vi "9401PWM with Midi.vi"() -> ()   [LabVIEW 2013]
panel:
  out "PWM1":dbl
  out "x .and. y?":bool
  out "error out 2":errorcluster
  out "duration (min:sec)":string="0:00"
  out "Text":string
  out "Track number: name [channel(s) used]":string="Please select a MIDI file..."
  in  "MIDI file (.mid)":path
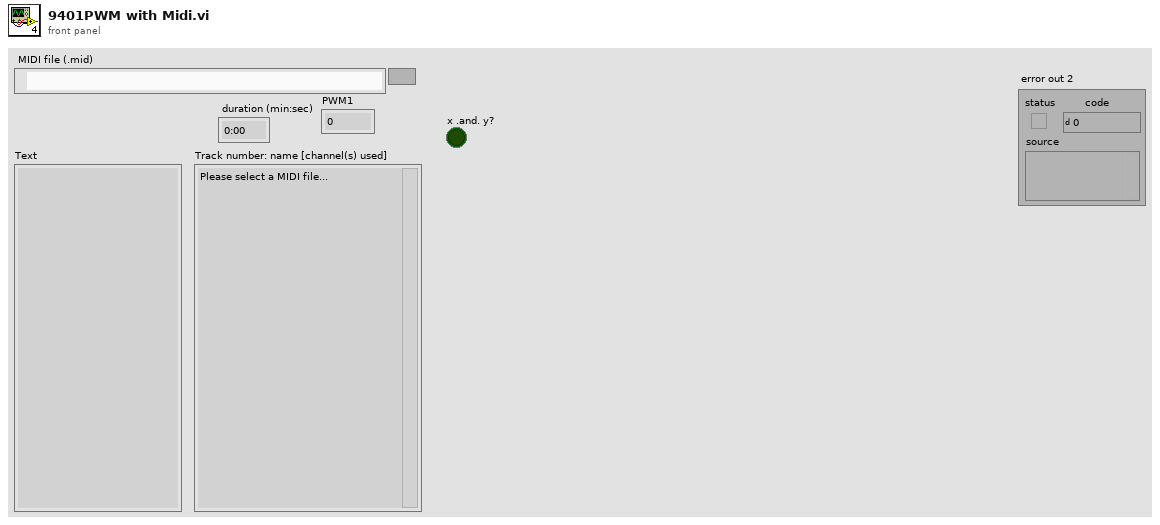
[diagram p1: front panel]
types:
  T1 = cluster{"type":u16, "tracks":u16, "ticks per qnote":u16}
  T2 = cluster{"note events":dbl[][], "duration [seconds]":dbl, "track info":string, "text meta-events":string}
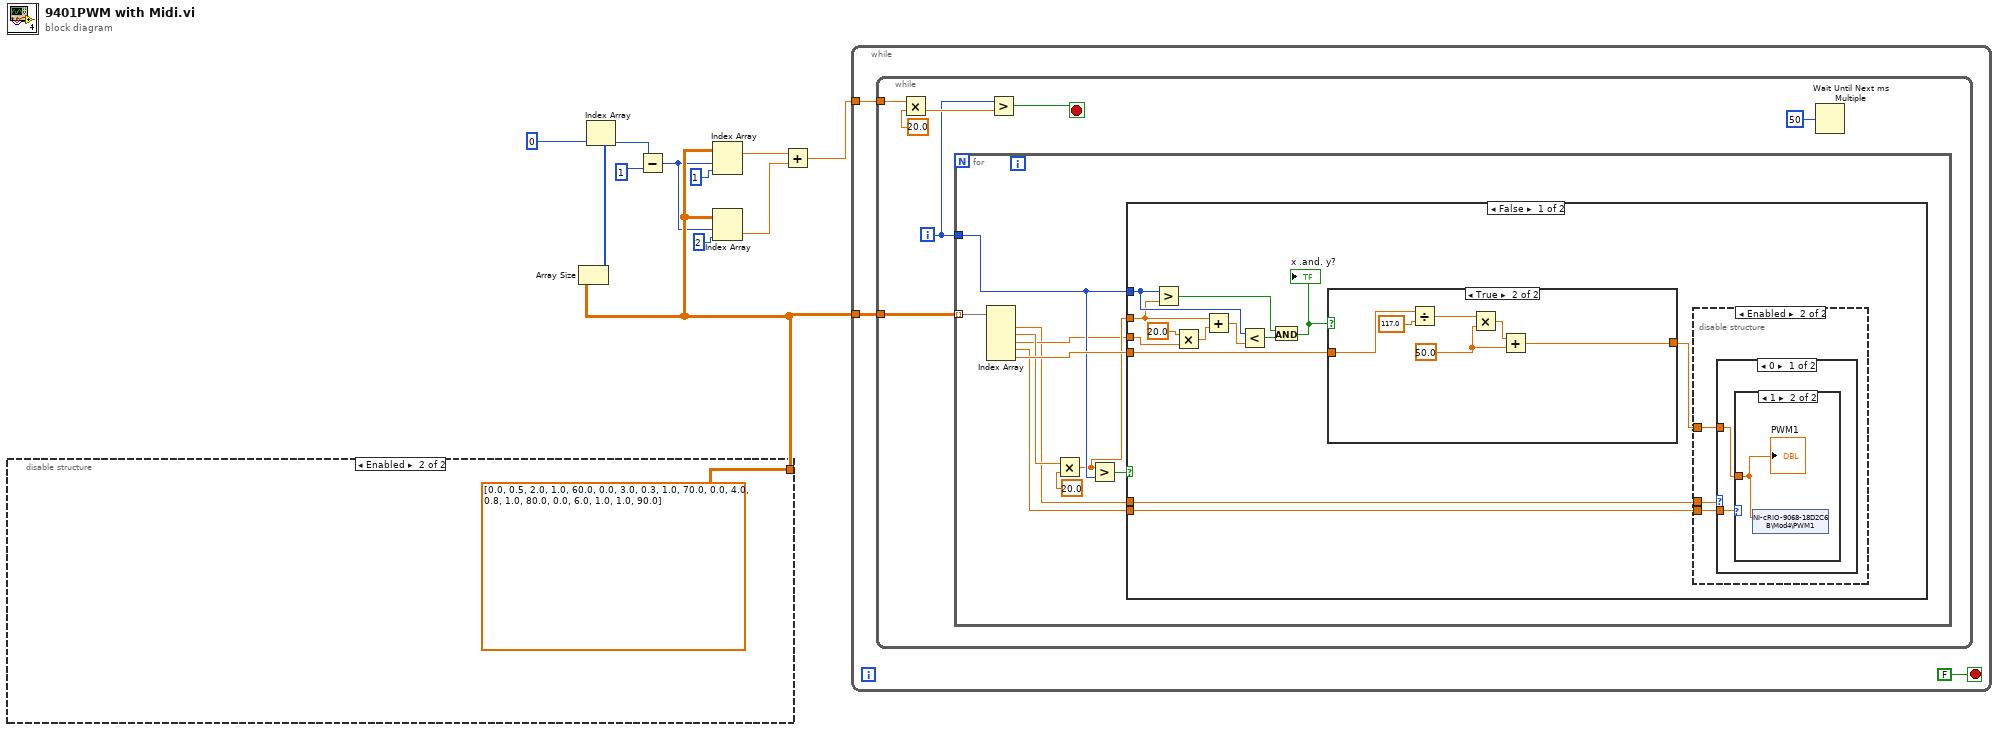
[diagram p0: block diagram]
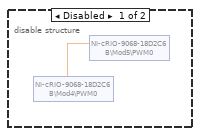
[diagram p2: hidden frame]
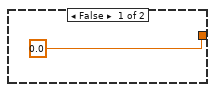
[diagram p5: hidden frame]
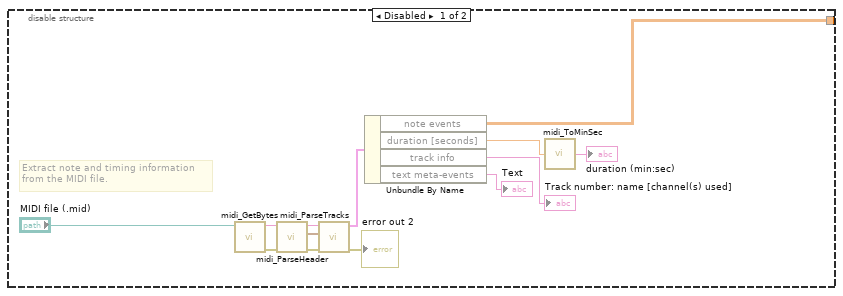
[diagram p7: hidden frame]
diagram:
  n1 = disable-structure shown="Enabled" {
    disable-tunnel: [w13 dbl[][] [[0.0, 0.5, 2.0, 1.0, 60.0], [0.0, 3.0, 0.3, 1.0, 70.0], [0.0, 4.0, 0.8, 1.0, 80.0], [0.0, 6.0, 1.0, 1.0, 90.0]] ("note events")] -> w6
    frame Disabled {
      # "Extract note and timing information\nfrom the MIDI file."
      n2 = call "midi_GetBytes.vi"("folder name"="MIDI file (.mid)") -> ("error out"=w14:errorcluster, "string"=w22:string)  [unwired: 8 in, 1 out]
      n3 = call "midi_ParseHeader.vi"("error in (no error)"=w14, "string in"=w22) -> ("error out"=w20:errorcluster, "header info"=w16:T1, "string out"=w21:string)  [unwired: 7 in]
      n4 = call "midi_ParseTracks.vi"("error in (no error)"=w20, "header info"=w16, "string in"=w21) -> ("error out"=→"error out 2":errorcluster, "file contents"=w19:T2)  [unwired: 7 in]
      n5 = Unbundle By Name(w19) -> ("note events"=w13:dbl[][], "duration [seconds]"=w15:dbl, "track info"=→"Track number: name [channel(s) used]":string, "text meta-events"=→"Text":string)
      n6 = call "midi_ToMinSec.vi"("seconds"=w15) -> ("min:sec"=→"duration (min:sec)":string)
    }
    frame Enabled {
    }
  }
  n7 = Array Size(array=w6) -> (size(s)=w11:i32[])
  n8 = Index Array(array=w11, index=0) -> (element=w8:i32)
  n9 = Subtract(x=w8, y=1) -> (x-y=w5:i32)
  n10 = Index Array(array=w6, index (row)=w5, index (col)=1 ("disabled index (col)")) -> (element=w2:dbl)
  n11 = Index Array(array=w6, index (row)=w5, index (col)=2 ("disabled index (col)")) -> (element=w1:dbl)
  n12 = Add(x=w2, y=w1) -> (x+y=w3:dbl)
  n13 = while {
    tunnel: w6 -> [w28]
    tunnel: w3 -> [w27]
    stop <- FALSE stop-if-true
    n14 = while {
      tunnel: w28 -> [w35]
      tunnel: w27 -> [w29]
      i -> [w30]
      stop <- w31 stop-if-true
      n15 = Multiply(x=w29, y=20.0) -> (x*y=w32:dbl)
      n16 = for {
        tunnel: w35 -> [w36] mode=indexing
        tunnel: w30 -> [w42]
        n17 = Index Array(array=w36) -> (element #1=w37:dbl, element #2=w43:dbl, element #3=w39:dbl, element #4=w38:dbl, element #5=w44:dbl)  [unwired: 5 in]
        n18 = Multiply(x=w43, y=20.0) -> (x*y=w40:dbl)
        n19 = Greater?(x=w40, y=w42) -> (0:w41:bool)
        n20 = case shown="False" w41 {
          tunnel: w44 -> [w58 _]
          tunnel: w42 -> [w51 _]
          tunnel: w40 -> [w50 _]
          tunnel: w39 -> [w52 _]
          tunnel: w38 -> [w49 _]
          tunnel: w37 -> [w48 _]
          frame False {
            n21 = Greater?(x=w51, y=w50) -> (0:w55:bool)
            n22 = Multiply(x=20.0, y=w52) -> (x*y=w56:dbl)
            n23 = Add(x=w50, y=w56) -> (x+y=w57:dbl)
            n24 = Less?(x=w51, y=w57) -> (x < y?=w54:bool)
            n25 = And(x=w55, y=w54) -> (x .and. y?=w47:bool)
            "x .and. y?" <- w47
            n26 = case shown="True" w47 {
              tunnel: w58 -> [_ w68]
              tunnel: [0.0 ("PWM0") w67] -> w46
              frame False {
              }
              frame True {
                w69 = 50.0 ("y")
                n27 = Divide(x=w68, y=117.0) -> (x/y=w71:dbl)
                n28 = Multiply(x=w71, y=w69) -> (x*y=w70:dbl)
                n29 = Add(x=w70, y=w69) -> (x+y=w67:dbl)
              }
            }
            n30 = disable-structure shown="Enabled" {
              disable-tunnel: w49 -> [_ w62]
              disable-tunnel: w48 -> [_ w61]
              disable-tunnel: w46 -> [_ w60]
              frame Disabled {
                n31 = shared-variable "NI-cRIO-9068-18D2C6B\\Mod5\\PWM0"() -> (w59:dbl)  [unwired: 1 in, 1 out]
                n32 = shared-variable "NI-cRIO-9068-18D2C6B\\Mod4\\PWM0"(w59) -> ()  [unwired: 1 in, 1 out]
              }
              frame Enabled {
                n33 = case shown="0" w61 {
                  tunnel: w62 -> [w64 _]
                  tunnel: w60 -> [w63 _]
                  frame 0 {
                    n34 = case shown="1" w64 {
                      tunnel: w63 -> [_ w65]
                      frame 0, Default {
                      }
                      frame 1 {
                        n35 = shared-variable "NI-cRIO-9068-18D2C6B\\Mod4\\PWM1"(w65) -> ()  [unwired: 1 in, 1 out]
                        "PWM1" <- w65
                      }
                    }
                  }
                  frame Default {
                  }
                }
              }
            }
          }
          frame True {
          }
        }
      }
      n36 = Greater?(x=w30, y=w32) -> (0:w31:bool)
      n37 = Wait Until Next ms Multiple(millisecond multiple=u32 50) -> ()  [unwired: 1 out]
    }
  }
